vi "Istwerte verarbeiten Alarme.vi"(8 "error in (no error)":errorcluster caption="Fehler (Eingang, kein Fehler)", 10 "Istwerte":u16[](array[numeric]), 11 "Schneider Steuerung PNS Eingang":refnum<class "Schneider Steuerung PNS.lvclass">) -> (0 "error out":errorcluster caption="Fehler (Ausgang)", 3 "Schneider Steuerung PNS Ausgang":refnum<class "Schneider Steuerung PNS.lvclass">)   [LabVIEW 2020, in "Schneider Steuerung PNS.lvclass"]
uses:
  Schneider Steuerung PNS.lvclass
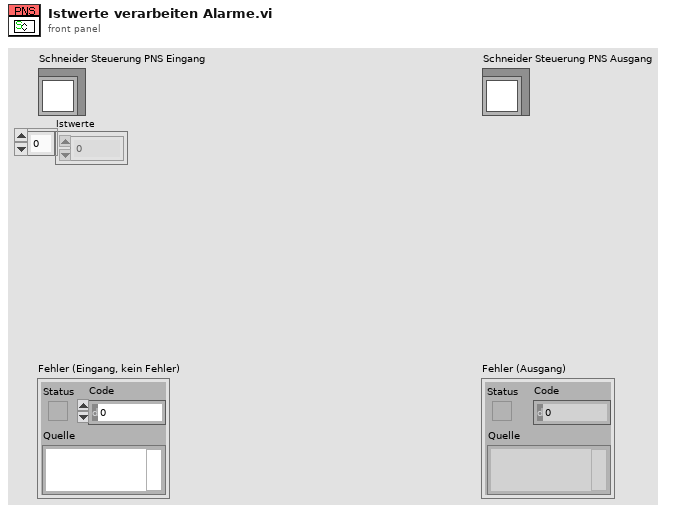
[diagram p1: front panel]
types:
  T1 = cluster{"Istwerte[0]":u16, "Istwerte[1]":u16, "Istwerte[2]":u16, "Istwerte[3]":u16, "Istwerte[4]":u16, "Istwerte[5]":u16, "Istwerte[6]":u16, "Istwerte[7]":u16, "Istwerte[8]":u16, "Istwerte[9]":u16, "Istwerte[10]":u16, "Istwerte[11]":u16, "Istwerte[12]":u16, "Istwerte[13]":u16, "Istwerte[14]":u16, "Istwerte[15]":u16}
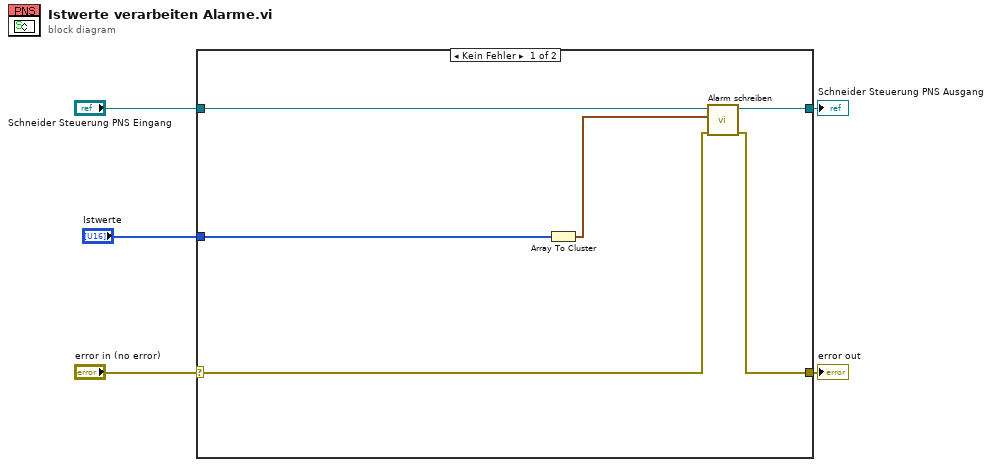
[diagram p0: block diagram]
diagram:
  n1 = case shown="Kein Fehler" "error in (no error)" {
    selector: "error in (no error)" -> [w7 w13]
    tunnel: [w6 w13] -> w4
    tunnel: [w9 w12] -> w2
    tunnel: "Schneider Steuerung PNS Eingang" -> [w11 w12]
    tunnel: "Istwerte" -> [w10 _]
    frame No Error {
      n2 = Array To Cluster(array=w10) -> (cluster=w8:T1)
      n3 = call-dynamic "Alarm schreiben.vi"("error in (no error)"=w7, "Alarm"=w8, "Steuerung PNS (Eingang)"=w11) -> ("error out"=w6:errorcluster, "Steuerung PNS (Ausgang)"=w9:refnum<class "Schneider Steuerung PNS.lvclass">)  [unwired: 7 in]
    }
    frame Error {
    }
  }
  "error out" <- w4
  "Schneider Steuerung PNS Ausgang" <- w2
